vi "Apply Tombstone Target.vi"   [LabVIEW 2017, in "Tests.lvlib" / "Toolkit.lvlib"]
uses:
  Toolkit.lvlib
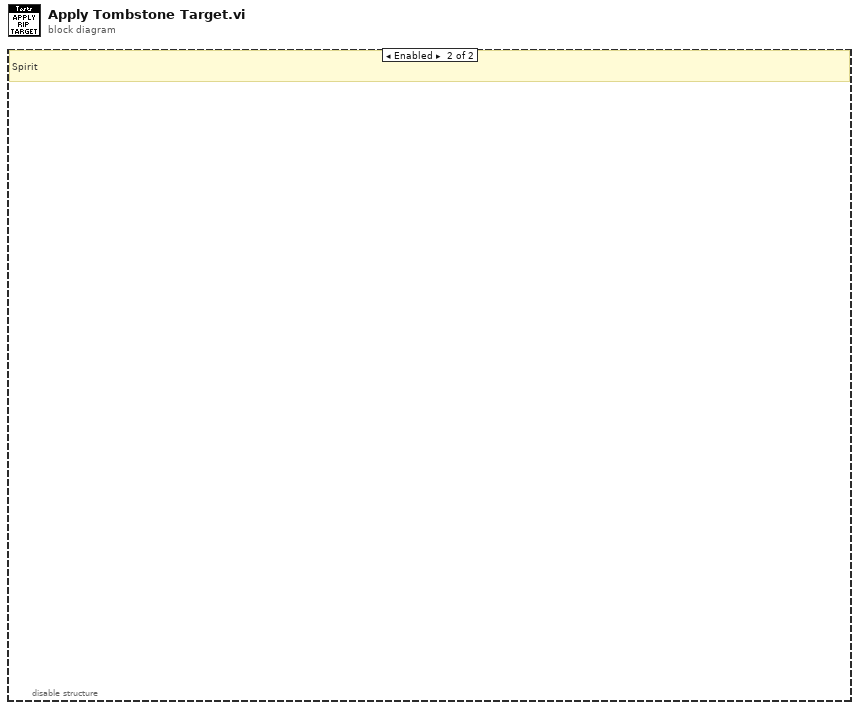
[diagram p0: block diagram]
diagram:
  n1 = disable-structure shown="Enabled" {
    frame Disabled {
      # "Corpse"
    }
    frame Enabled {
      # "Spirit"
    }
  }
